vi "Increment.vi"(8 "error in (no error)":errorcluster, 11 "Complex in":refnum<class "Complex.lvclass">) -> (0 "error out":errorcluster, 3 "Complex out":refnum<class "Complex.lvclass">)   [LabVIEW 2020, in "Complex.lvclass"]
uses:
  Complex.lvclass
  Counter/Counter.lvclass
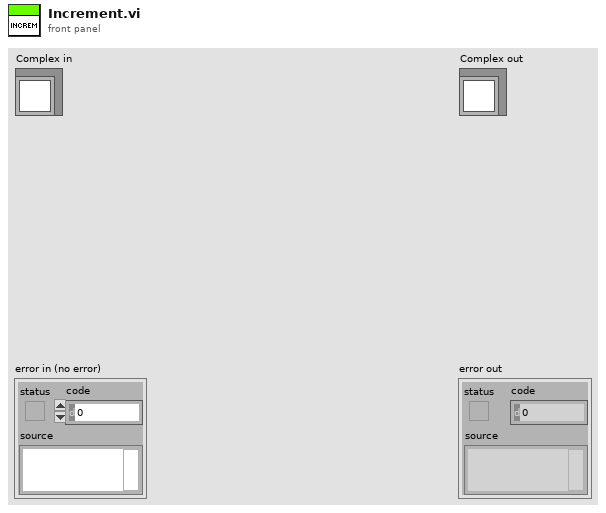
[diagram p1: front panel]
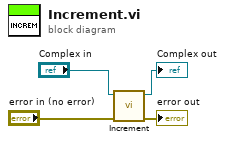
[diagram p0: block diagram]
diagram:
  n1 = call-parent "Increment.vi"("error in (no error)"="error in (no error)", "Counter in"="Complex in") -> ("error out"=→"error out":errorcluster, "Counter out"=→"Complex out":refnum<class "Complex.lvclass">)  [unwired: 8 in]
